vi "Register.vi"(8 "error in":errorcluster, 11 "Data":refnum<class "Data.lvclass">) -> (0 "error out":errorcluster)   [LabVIEW 2020, in "Data.lvclass"]
uses:
  Data.lvclass
  Data.lvclass/Data.ctl
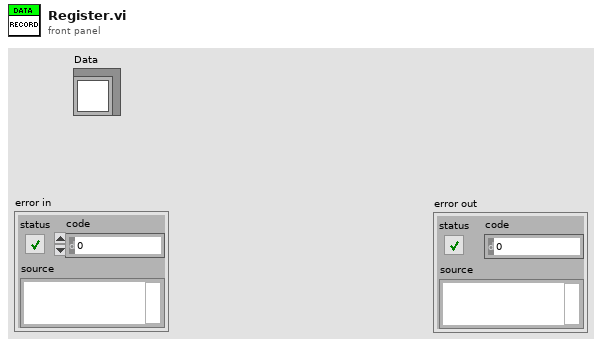
[diagram p1: front panel]
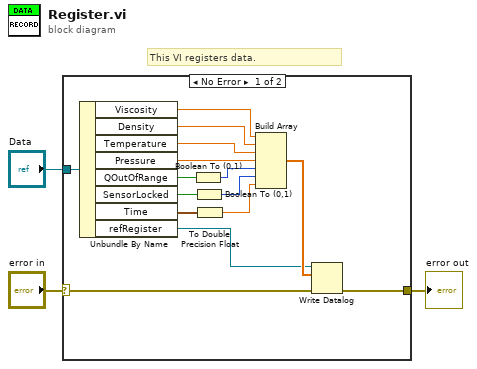
[diagram p0: block diagram]
diagram:
  # "This VI registers data."
  n1 = case shown="No Error" "error in" {
    selector: "error in" -> [w5 w19]
    tunnel: "Data" -> [w18 _]
    tunnel: [w4 w19] -> w1
    frame No Error {
      n2 = Unbundle By Name(w18) -> ("Viscosity"=w14:dbl, "Density"=w13:dbl, "Temperature"=w12:dbl, "Pressure"=w11:dbl, "QOutOfRange"=w17:bool, "SensorLocked"=w16:bool, "Time"=w15:timestamp, "refRegister"=w6:refnum<k1>)
      n3 = Boolean To (0,1)(Boolean=w17) -> (0, 1=w10:i16)
      n4 = Boolean To (0,1)(Boolean=w16) -> (0, 1=w9:i16)
      n5 = To Double Precision Float(number=w15) -> (double precision float=w8:dbl)
      n6 = Build Array(w14, w13, w12, w11, w10, w9, w8) -> (w7:dbl[])
      n7 = Write Datalog(4:w5, 6:w7, 7:w6) -> (0:w4:errorcluster)  [unwired: 1 out]
    }
    frame Error {
    }
  }
  "error out" <- w1
